vi "Get.vi"(11 "ID in":refnum<class "ID.lvclass">) -> (2 "Entity ID":T1)   [LabVIEW 2020, in "Conditum.lvlib" / "Columns.lvlib" / "ID.lvclass"]
uses:
  ID.lvclass
  Entity ID.ctl
  Conditum.lvlib
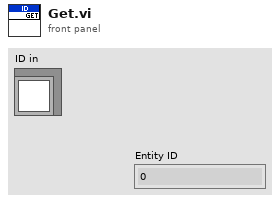
[diagram p1: front panel]
types:
  T1 = typedef "Conditum.lvlib/Entity ID.ctl" = i64
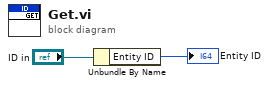
[diagram p0: block diagram]
diagram:
  n1 = Unbundle By Name("ID in") -> ("Entity ID"=→"Entity ID":T1)
